vi "Exp Random Lab.vi"() -> ()   [LabVIEW 2010]
uses:
  <vilib>/Utility/file.llb/Write To Spreadsheet File (DBL).vi
  <vilib>/Analysis/NI_AALBase.lvlib
panel:
  in  "Histogram intervals":i32=10
  out "Histogram":T1(graph)
  in  "How many random numbers?":i32
  in  "How many desired expected random numbers?":dbl
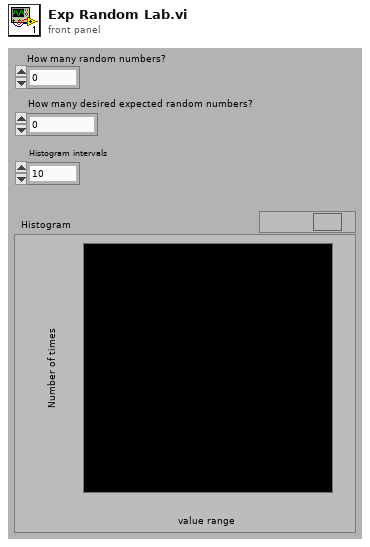
[diagram p1: front panel]
types:
  T1 = cluster{"X Values":dbl[], "Histogram: h(x)":i32[]}
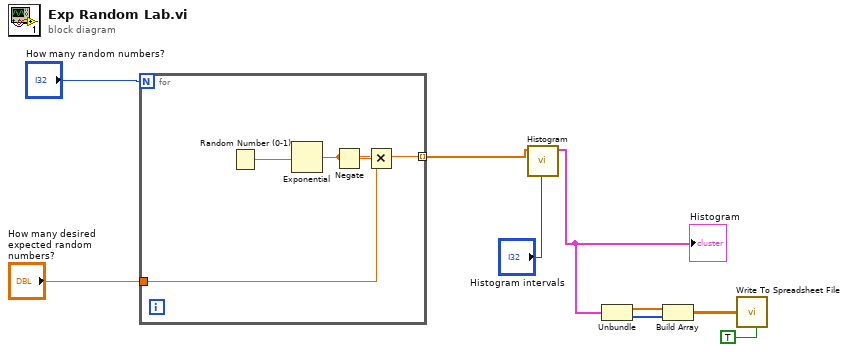
[diagram p0: block diagram]
diagram:
  n1 = for {
    N: "How many random numbers?" -> [_]
    tunnel: [w10] -> w1 mode=indexing
    tunnel: "How many desired expected random numbers?" -> [w12]
    n2 = Random Number (0-1)() -> (number: 0 to 1=w11:dbl)
    n3 = Exponential(1:w11) -> (0:w10:dbl)
    n4 = Negate(x=w10) -> (-x=w13:dbl)
    n5 = Multiply(x=w13, y=w12) -> ()  [unwired: 1 out]
  }
  n6 = call <vilib>:"Histogram.vi"("intervals"="Histogram intervals", "X"=w1) -> ("Histogram Graph"=w6:T1)  [unwired: 6 in, 3 out]
  "Histogram" <- w6
  n7 = Unbundle(w6) -> ("X Values"=w5:dbl[], "Histogram: h(x)"=w4:i32[])
  n8 = Build Array(w5, w4) -> (w3:dbl[][])
  n9 = call-poly <vilib>:"Write To Spreadsheet File.vi"("transpose? (no:F)"=TRUE, "2D data"=w3) -> ()  [unwired: 6 in, 1 out]
